vi "Cp-Cpk-Calculation.vi"(7 "Zen Analytics in":refnum<class "Zen Analytics.lvclass">, 8 "error in (no error)":errorcluster, 10 "Graph Refference's":T1, 11 "Statistical params":string[][](array[string])) -> (0 "error out":errorcluster)   [LabVIEW 2019, in "Zen Analytics.lvlib" / "Zen Analytics.lvclass"]
uses:
  Zen Analytics.lvclass
  Dependency/GraphReff.ctl
  <vilib>/ActorFramework/Message Enqueuer/Message Enqueuer.lvclass
  Dependency/AnalyticsDataToSM.ctl
types:
  T1 = typedef "Zen Analytics.lvlib/Zen Analytics.lvclass/GraphReff.ctl" = cluster{"HistgramGraph-reff":refnum<vi>[], "BarGraph-reff":refnum<vi>[], "PieGraph-reff":refnum<vi>[], "Lable-reff":refnum<vi>[], "TrendGraph-reff":refnum<vi>[], "CpCpkTable":refnum<vi>}
  T2 = typedef "Zen Analytics.lvlib/Zen Analytics.lvclass/AnalyticsDataToSM.ctl" = cluster{"Actor Info":cluster{"Analytics Enqueuer":refnum<class "Message Enqueuer.lvclass">, "This VI":refnum<vi>, "Module name":string}, "Statistical Info":string[][], "Graph Refference's":T1, "ErrorMessage":string}
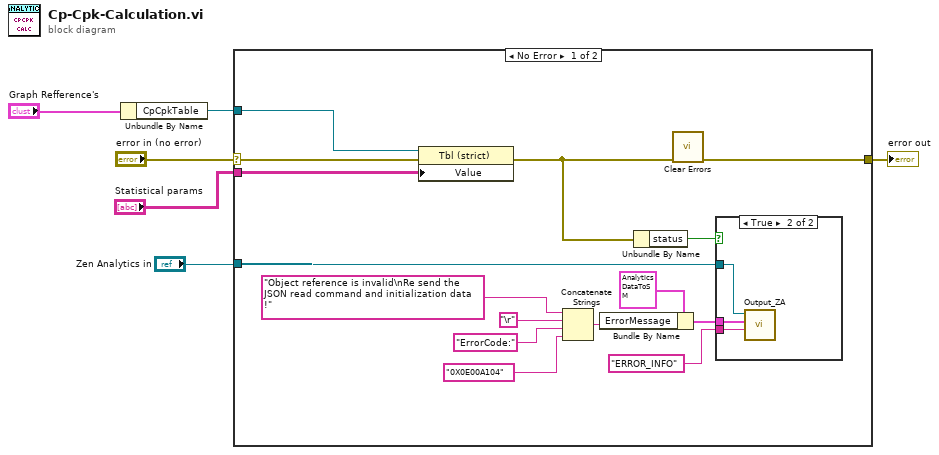
[diagram p0: block diagram]
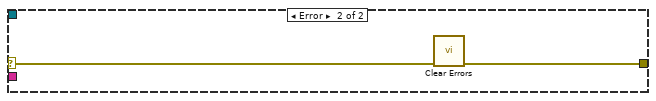
[diagram p3: hidden frame]
diagram:
  n1 = Unbundle By Name("Graph Refference's") -> ("CpCpkTable"=w3:refnum<vi>)
  n2 = case shown="No Error" "error in (no error)" {
    selector: "error in (no error)" -> [w19 w26]
    tunnel: [w9 w25] -> w5
    tunnel: w3 -> [w21 _]
    tunnel: "Statistical params" -> [w20 _]
    tunnel: "Zen Analytics in" -> [w10 _]
    frame No Error {
      n3 = property class="Tbl (strict)"(reference=w21, error in=w19, "Value"=w20) -> (error out=w11:errorcluster)  [unwired: 1 out]
      n4 = Concatenate Strings("Object reference is invalid\nRe send the JSON read command and initialization data !" ("SolutionForError"), "\r", "ErrorCode:", "0X0E00A104" ("ErrorCode")) -> (w12:string)
      n5 = Bundle By Name(cluster=T2 {"Actor Info"={"Analytics Enqueuer"=refnum, "This VI"=refnum, "Module name"=""}, "Statistical Info"=[], "Graph Refference's"={"HistgramGraph-reff"=[], "BarGraph-reff"=[], "PieGraph-reff"=[], "Lable-reff"=[], "TrendGraph-reff"=[], "CpCpkTable"=refnum}, "ErrorMessage"=""} ("Analytics Information"), "ErrorMessage"=w12) -> (w15:T2)
      n6 = Unbundle By Name(w11) -> ("status"=w18:bool)
      n7 = call <vilib>:"Clear Errors.vi"("error in (no error)"=w11) -> ("error out"=w9:errorcluster)  [unwired: 5 in, 1 out]
      n8 = case shown="True" w18 {
        tunnel: "ERROR_INFO" ("State") -> [_ w24]
        tunnel: w10 -> [_ w23]
        tunnel: w15 -> [_ w22]
        frame False {
        }
        frame True {
          n9 = call "Output_ZA.vi"("State"=w24, "Analytics Information"=w22, "Zen Analytics in"=w23) -> ()  [unwired: 7 in, 2 out]
        }
      }
    }
    frame Error {
      n10 = call <vilib>:"Clear Errors.vi"("error in (no error)"=w26) -> ("error out"=w25:errorcluster)  [unwired: 5 in, 1 out]
    }
  }
  "error out" <- w5
